vi "Blink FGV Tester.vi"() -> ()   [LabVIEW 2015]
panel:
  in  "Unblink Button":bool
  in  "Stop Button":bool
  in  "Blink Button":bool
  in  "String":string
  in  "Numeric Control":dbl
  in  "Boolean":bool
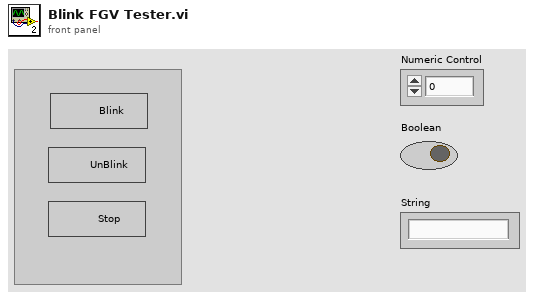
[diagram p1: front panel]
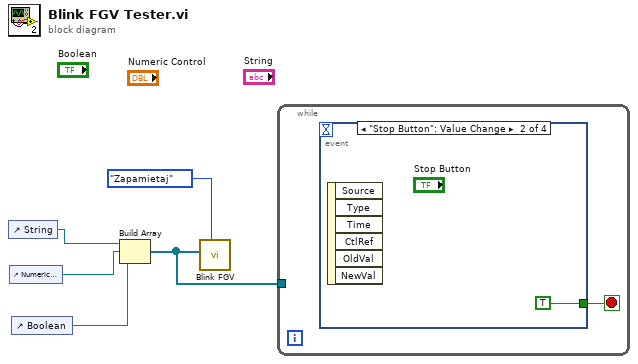
[diagram p0: block diagram]
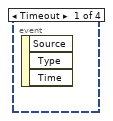
[diagram p2: hidden frame]
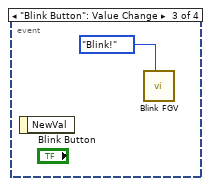
[diagram p3: hidden frame]
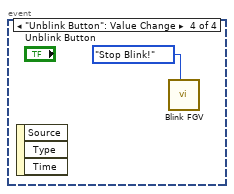
[diagram p4: hidden frame]
diagram:
  n1 = control-ref of="String"() -> (w4:refnum<vi>)
  n2 = control-ref of="Numeric Control"() -> (w3:refnum<vi>)
  n3 = control-ref of="Boolean"() -> (w2:refnum<vi>)
  n4 = Build Array(w4, w3, w2) -> (w1:refnum<vi>[])
  n5 = call "Blink FGV.vi"("Akcja"=enum16{"Zapamietaj", "Blink!", "Stop Blink!"}."Zapamietaj", "Referencje"=w1) -> ()  [unwired: 10 in]
  n6 = while {
    tunnel: w1 -> [_]
    stop <- w6 stop-if-true
    n7 = event shown="[1] \"Stop Button\": Value Change" {
      selector: _ -> [_ _ _ _]
      dyn-events: _ -> [_ _ _ _]
      timeout: _ -> [_ _ _ _]
      tunnel: [_ TRUE _ _] -> w6
      event Timeout {
        n8 = event-data() -> ()  [unwired: 1 in, 3 out]
      }
      event "Stop Button": Value Change {
        n9 = event-data() -> ()  [unwired: 1 in, 6 out]
      }
      event "Blink Button": Value Change {
        n10 = event-data() -> ()  [unwired: 1 in, 1 out]
        n11 = call "Blink FGV.vi"("Akcja"=enum16{"Zapamietaj", "Blink!", "Stop Blink!"}."Blink!") -> ()  [unwired: 11 in]
      }
      event "Unblink Button": Value Change {
        n12 = event-data() -> ()  [unwired: 1 in, 3 out]
        n13 = call "Blink FGV.vi"("Akcja"=enum16{"Zapamietaj", "Blink!", "Stop Blink!"}."Stop Blink!") -> ()  [unwired: 11 in]
      }
    }
  }
